vi "Wrap Image Dat.vi"(8 "error in (no error)":errorcluster, 9 "is canceled?":bool, 10 "Array":u16[](array[numeric]), 11 "Measure Call Context in":refnum<class "Measure Call Context.lvclass">) -> (0 "error out":errorcluster)   [LabVIEW 2025, in "GettingStarted_Common_148X_Host.lvlib"]
uses:
  1487 HIHO GSE/Host/Common/GettingStarted_Common_148X_Host.lvlib
  <vilib>/Plug-In SDKs/Measurements/Measure Call Context/Measure Call Context.lvclass
  Measurement Results.ctl
  Automotive Vision.lvclass
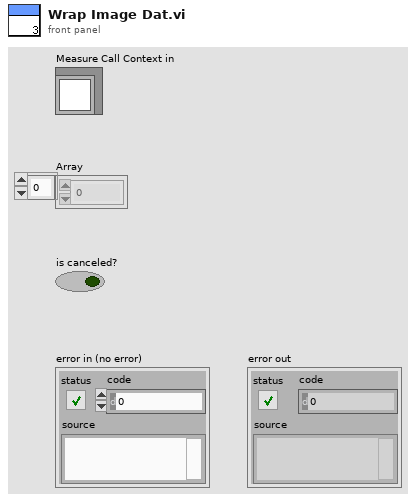
[diagram p1: front panel]
types:
  T1 = typedef "Automotive Vision.lvclass/Measurement Results.ctl" = cluster{"ACQ. IN PROGRESS":bool, "Array":u32[]}
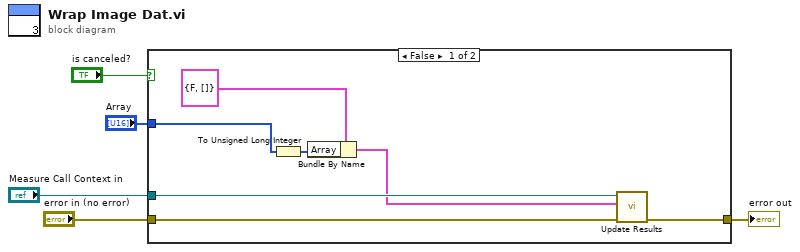
[diagram p0: block diagram]
diagram:
  n1 = case shown="False" "is canceled?" {
    tunnel: "error in (no error)" -> [w12 w13]
    tunnel: [w11 w13] -> w3
    tunnel: "Measure Call Context in" -> [w10 _]
    tunnel: "Array" -> [w7 _]
    frame False {
      n2 = To Unsigned Long Integer(number=w7) -> (unsigned 32bit integer=w6:u32[])
      n3 = Bundle By Name(cluster=T1 {"ACQ. IN PROGRESS"=FALSE, "Array"=[]} ("measurement results"), "Array"=w6) -> (w8:T1)
      n4 = call <vilib>:"Update Results.vi"("error in"=w12, "measurement results"=w8, "measure call context in"=w10) -> ("error out"=w11:errorcluster)  [unwired: 7 in, 1 out]
    }
    frame True {
    }
  }
  "error out" <- w3
